vi "data logging.vi"(1 "Part1 2":string, 2 "Part1":string) -> (0 "Output String":string)   [LabVIEW 2009]
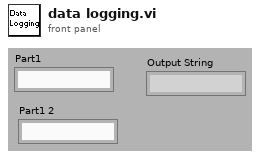
[diagram p1: front panel]
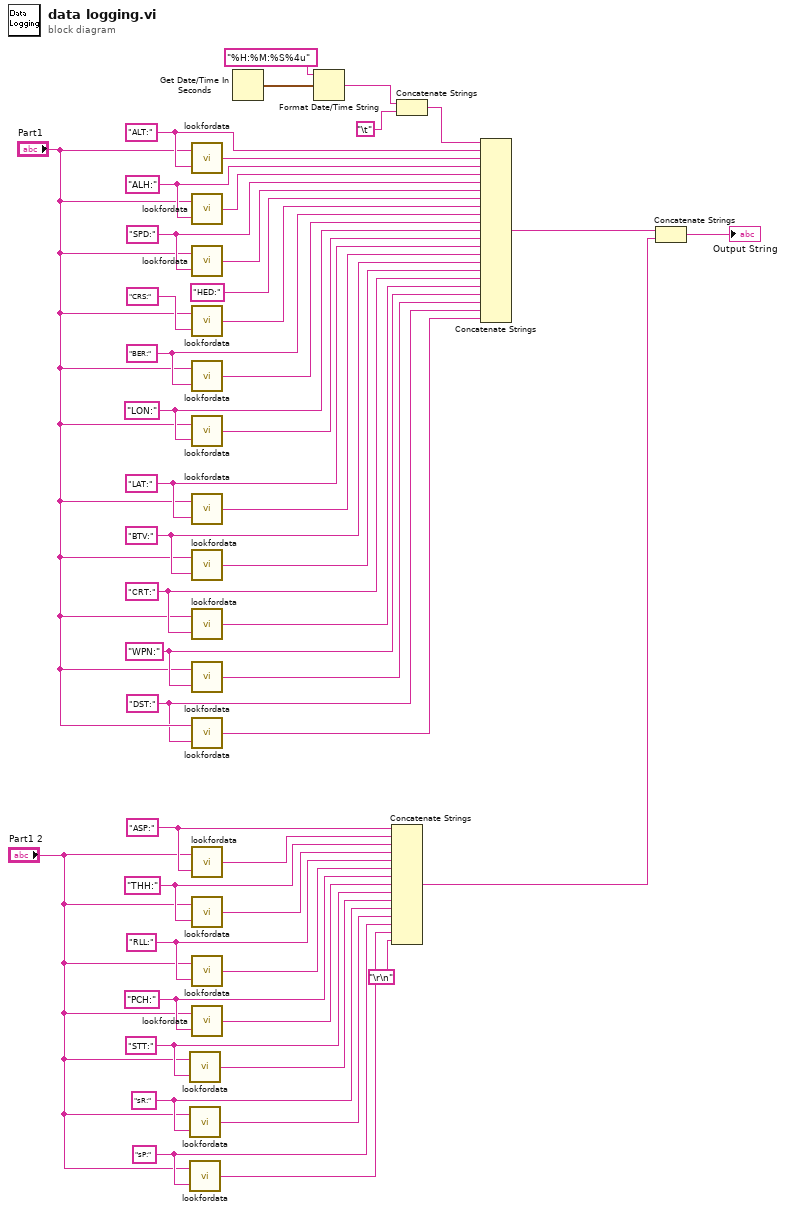
[diagram p0: block diagram]
diagram:
  w4 = "sP:" ("Header")
  w6 = "sR:" ("Header")
  w8 = "STT:" ("Header")
  w16 = "PCH:" ("Header")
  w18 = "RLL:" ("Header")
  w20 = "THH:" ("regular expression")
  w22 = "ASP:" ("regular expression")
  w32 = "BTV:" ("Header")
  w29 = "CRT:" ("Header")
  w34 = "LAT:" ("Header")
  w36 = "LON:" ("Header")
  w42 = "SPD:" ("Header")
  w25 = "DST:" ("Header")
  w27 = "WPN:" ("Header")
  w38 = "BER:" ("Header")
  w44 = "ALH:" ("regular expression")
  w45 = "ALT:" ("regular expression")
  n1 = call "lookfordata.vi"("Header"=w8, "string"="Part1 2") -> ("output string"=w7:string)
  n2 = call "lookfordata.vi"("Header"=w6, "string"="Part1 2") -> ("output string"=w5:string)
  n3 = call "lookfordata.vi"("Header"=w4, "string"="Part1 2") -> ("output string"=w3:string)
  n4 = call "lookfordata.vi"("Header"=w45, "string"="Part1") -> ("output string"=w46:string)
  n5 = call "lookfordata.vi"("Header"=w44, "string"="Part1") -> ("output string"=w43:string)
  n6 = call "lookfordata.vi"("Header"=w42, "string"="Part1") -> ("output string"=w41:string)
  n7 = call "lookfordata.vi"("Header"="CRS:", "string"="Part1") -> ("output string"=w40:string)
  n8 = call "lookfordata.vi"("Header"=w38, "string"="Part1") -> ("output string"=w37:string)
  n9 = call "lookfordata.vi"("Header"=w36, "string"="Part1") -> ("output string"=w35:string)
  n10 = call "lookfordata.vi"("Header"=w34, "string"="Part1") -> ("output string"=w33:string)
  n11 = call "lookfordata.vi"("Header"=w32, "string"="Part1") -> ("output string"=w31:string)
  n12 = call "lookfordata.vi"("Header"=w29, "string"="Part1") -> ("output string"=w30:string)
  n13 = call "lookfordata.vi"("Header"=w27, "string"="Part1") -> ("output string"=w28:string)
  n14 = call "lookfordata.vi"("Header"=w25, "string"="Part1") -> ("output string"=w24:string)
  n15 = call "lookfordata.vi"("Header"=w22, "string"="Part1 2") -> ("output string"=w23:string)
  n16 = call "lookfordata.vi"("Header"=w20, "string"="Part1 2") -> ("output string"=w21:string)
  n17 = call "lookfordata.vi"("Header"=w18, "string"="Part1 2") -> ("output string"=w19:string)
  n18 = call "lookfordata.vi"("Header"=w16, "string"="Part1 2") -> ("output string"=w17:string)
  n19 = Get Date/Time In Seconds() -> (seconds since 1Jan1904=w47:timestamp)
  n20 = Format Date/Time String(time format string (%c)="%H:%M:%S%4u", seconds (now)=w47) -> (date/time string=w11:string)  [unwired: 1 out]
  n21 = Concatenate Strings(w22, w23, w20, w21, w18, w19, w16, w17, w8, w7, w6, w5, w4, w3, "\r\n") -> (w15:string)
  n22 = Concatenate Strings(w11, "\t") -> (w10:string)
  n23 = Concatenate Strings(w10, w45, w46, w44, w43, w42, w41, "HED:" ("Header"), w40, w38, w37, w36, w35, w34, w33, w32, w31, w29, w30, w27, w28, w25, w24) -> (w14:string)
  n24 = Concatenate Strings(w14, w15) -> (→"Output String":string)
